vi "Write myRIO Data to the PI System via OMF (v1.0).vi"() -> ()   [LabVIEW 2014]
uses:
  <vilib>/Platform/TimedLoop/XDataNode/timing_clust.ctl
  <vilib>/Platform/TimedLoop/XDataNode/nitl_modes.ctl
  <vilib>/Platform/TimedLoop/XDataNode/wakeup.ctl
  <vilib>/myRIO/Instrument Drivers/Onboard Devices/Accelerometer/typedefs/Accelerometer Reference.ctl
  <vilib>/myRIO/Common/Instrument Driver Framework/Utilities/typedefs/myRIO Generic Hardware Reference.ctl
  <vilib>/myRIO/Common/Instrument Driver Framework/Utilities/typedefs/Hardware Version Enum.ctl
  <vilib>/myRIO/Common/Instrument Driver Framework/Utilities/typedefs/myRIO v1.0 Reference.ctl
  <vilib>/myRIO/Common/Instrument Driver Framework/Utilities/typedefs/Generic FPGA Reference.ctl
  <vilib>/myRIO/Common/Instrument Driver Framework/myRIO v1.0/Accelerometer/typedefs/Accelerometer Channels List.ctl
  <vilib>/myRIO/Common/Instrument Driver Framework/myRIO v1.0/Accelerometer/typedefs/Accelerometer Channels Enum.ctl
  <vilib>/userdefined/High Color/nirio_resource_hc.ctl
  <vilib>/myRIO/Common/Instrument Driver Framework/Utilities/vis/Is FPGA Ref Available.vi
  <vilib>/myRIO/Common/Instrument Driver Framework/myRIO v1.0/Accelerometer/vis/myRIO v1.1 Open Accelerometer.vi
  <vilib>/myRIO/Instrument Drivers/Onboard Devices/Accelerometer/vis/Read.vi
  <vilib>/myRIO/Common/Instrument Driver Framework/Utilities/vis/Validate Channels.vi
  <vilib>/myRIO/Common/Instrument Driver Framework/myRIO v1.0/Accelerometer/vis/myRIO v1.0 Reserve Accelerometer.vi
  <vilib>/myRIO/Common/Instrument Driver Framework/myRIO v1.0/Resource Manager/vis/myRIO v1.0 Reserve Channel List.vi
  <vilib>/myRIO/Common/Instrument Driver Framework/myRIO v1.0/Accelerometer/vis/myRIO v1.0 Build MUX Configuration Accelerometer.vi
  <vilib>/myRIO/Common/Instrument Driver Framework/myRIO v1.0/Resource Manager/vis/myRIO v1.0 Reserve Channel.vi
  <vilib>/myRIO/Common/Instrument Driver Framework/myRIO v1.0/Resource Manager/vis/myRIO v1.0 Unreserve Channel.vi
  <vilib>/myRIO/Common/Instrument Driver Framework/myRIO v1.0/Resource Manager/vis/myRIO v1.0 Build Mutex Name.vi
  <vilib>/Utility/VariantDataType/GetNumericInfo.vi
  <vilib>/Utility/error.llb/Error Cluster From Error Code.vi
  <vilib>/myRIO/Common/Instrument Driver Framework/myRIO v1.0/myRIO v1.1 Open.vi
  <vilib>/myRIO/Common/Instrument Driver Framework/myRIO v1.0/Accelerometer/vis/myRIO v1.0 Get Scaling Constant Accelerometer.vi
  <vilib>/myRIO/Common/Instrument Driver Framework/Utilities/vis/IO Manager.vi
  <vilib>/myRIO/Common/Instrument Driver Framework/Utilities/vis/Configuration Manager.vi
  <vilib>/myRIO/Common/Instrument Driver Framework/myRIO v1.0/myRIO v1.0 Close.vi
  <vilib>/myRIO/Common/Instrument Driver Framework/myRIO v1.0/Accelerometer/vis/myRIO v1.0 Read Accelerometer.vi
  <vilib>/platform/TimedLoop/XDataNode/XDataNode.xnode
  <vilib>/myRIO/Express VI/Onboard Devices/Accelerometer/Accelerometer Express VI.xnode
  <vilib>/myRIO/Instrument Drivers/Onboard Devices/Accelerometer/vis/myRIO Accelerometer Open.xnode
  <vilib>/Platform/TimedLoop/XDataNode/XDNodeRunTimeDep.lvlib
  <vilib>/myRIO/Instrument Drivers/Onboard Devices/Accelerometer/Accelerometer.lvlib
panel:
  out "Acceleration":T1(graph)
  in  "Stop looping":bool
  in  "OMF Static Type Instance Name":string="LabVIEW myRIO AF Element 3"
  out "Response body for initial OMF messages":string
  out "Reponse headers for initial OMF messages":string
  out "Number of continuous OMF data messages sent":i32
  out "Reponse body for continuous OMF data messages":string
  out "Response headers for continuous OMF data messages":string
  out "error out":errorcluster
  in  "Allow untrusted certificates?":bool=TRUE
  in  "OMF Dynamic Type Property Names and Formats":T2(array[cluster])=[{"Dynamic Property Name"="X acceleration", "Dynamic Property Format"=enum."number"}, {"Dynamic Property Name"="Y acceleration", "Dynamic Property Format"=enum."number"}, {"Dynamic Property Name"="Z acceleration", "Dynamic Property Format"=enum."number"}]
  in  "OMF Static Type Property Names, Formats, and Values":T3(array[cluster])=[{"Static Property Name"="Data ingress method", "Static Property Format"=enum."string", "Static Property Value"="\"OMF\""}]
  in  "Seconds in between continuous data messages":i32=1
  in  "OMF Static Type ID":string="LabVIEW myRIO Static Type 3"
  in  "OMF Dynamic Type ID":string="LabVIEW myRIO Dynamic Type 3"
  in  "OMF Container ID":string="LabVIEW myRIO Data Container 3"
  in  "OMF Producer Token":string="uid=034956ae-830c-4627-9778-e6724debe14b&crt=20180727152305511&sig=2y1S5b1wiy+iAvDMgQvLHble8CC54d+4WAt9WWHkGM8="
  in  "OMF Ingress URL":string="https://lopezpiserver:8118/ingress/messages"
  # "myRIO Accelerometer Data"
  # "Configuration"
  # "Response Messages"
  # "Note: if the response header is \"HTTP/1.1 204 No Content\" and the response body is empty, that indicates that a message was received successfully!"
  # "Note: the OMF Ingress URL and OMF Producer Token can be obtained from within the PI Data Collection Manager"
  # "(Stop sending continuous messages)"
  # "Note: If you are testing against a stock installation, one that still uses an untructed, self-signed certificate (which is the default), set this to \"ON\""
  # "Note: the Static Type Instance Name (below) will be the name of the PI AF Element that is created on the target PI System"
  # "Error Messages"
  # "Note: when specifying the value for a static property (above), if the property format is \"string\" add double quotes around the string value; if the property format \"number\", do not add double quotes around the numeric value."
  # "Note: remember the order in which you specify these dynamic properties! Later within your VI, you will wire in a string array of live data values for these dynamic properties, and the order of values in that array must match the order of properties that you specify above (i.e., if you listed that the first property is \"X acceleration\", you need to make sure that the first value in your string array is the x acceleration value)."
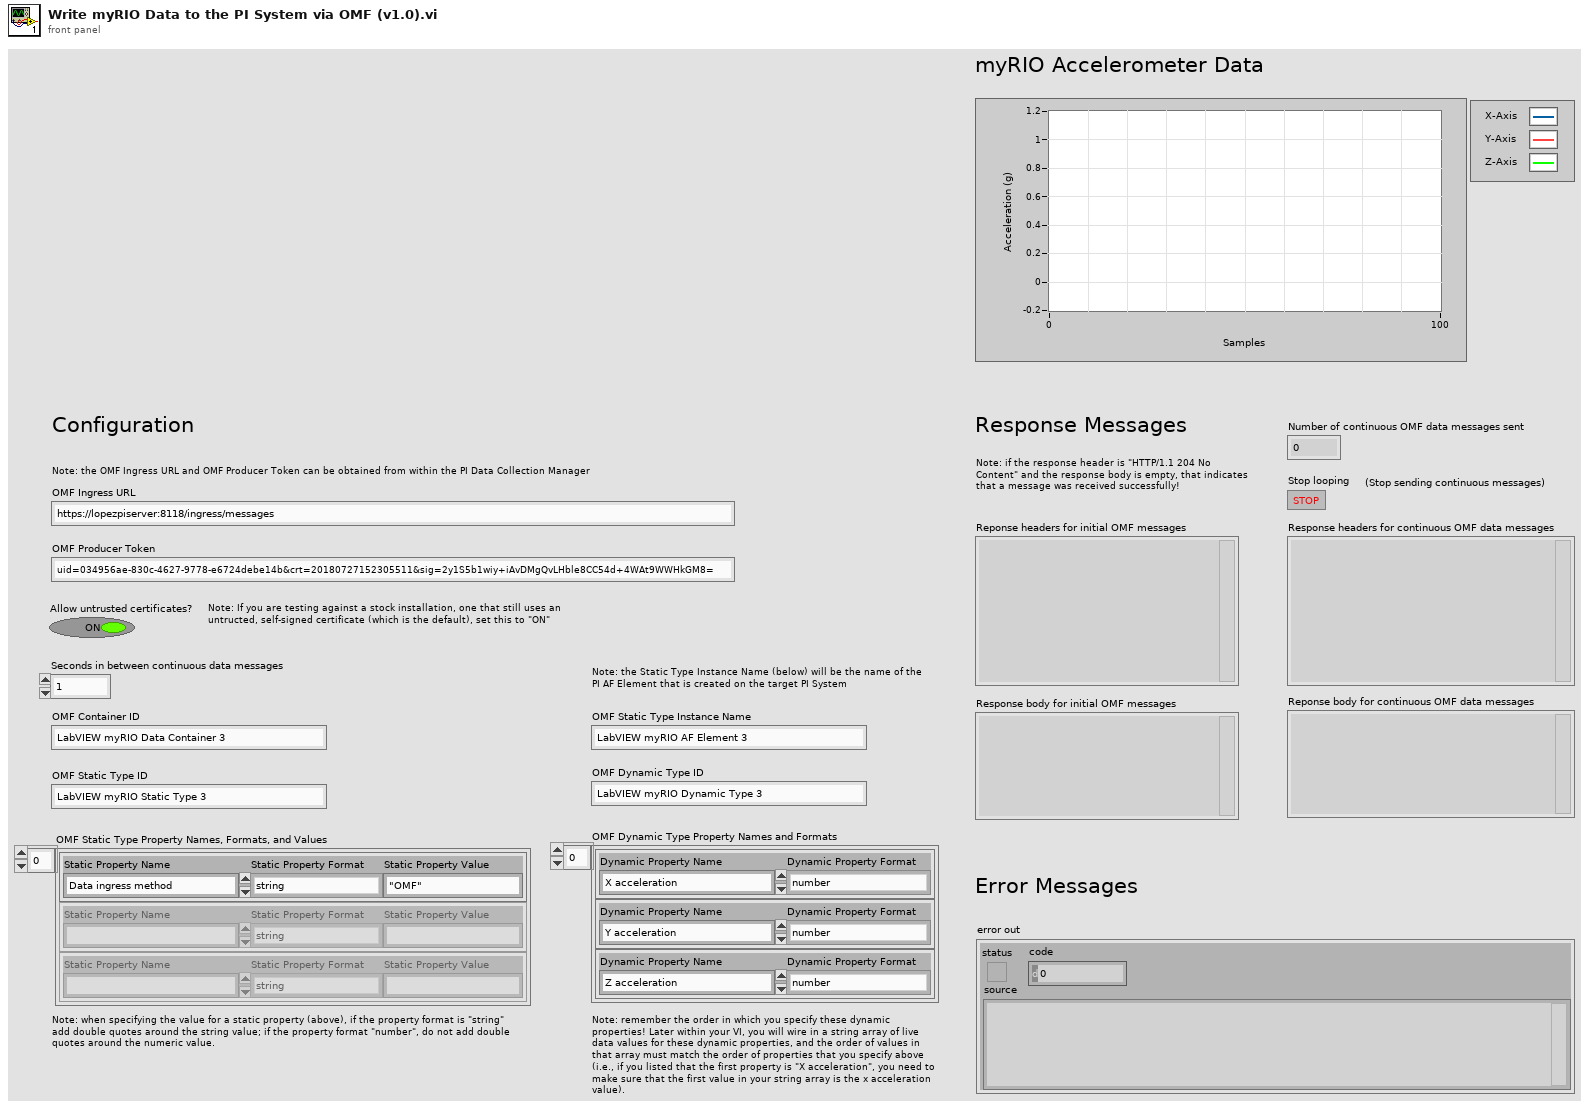
[diagram p1: front panel]
types:
  T1 = cluster{"X-Axis":dbl, "Y-Axis":dbl, "Z-Axis":dbl}
  T2 = cluster{"Dynamic Property Name":string, "Dynamic Property Format":enum16{"string", "number"}}[]
  T3 = cluster{"Static Property Name":string, "Static Property Format":enum16{"string", "number"}, "Static Property Value":string}[]
  T4 = typedef "LabVIEWHTTPClient.lvlib/ClientHandle.ctl" = refnum<k1>
  T5 = typedef "XDNodeRunTimeDep.lvlib/timing_clust.ctl" = cluster{"Expected End [f-1]":u64, "Actual End [f-1]":u64, "Finished Late? [f-1]":bool, "Expected End [i-1]":u64, "Actual End [i-1]":u64, "Finished Late? [i-1]":bool, "Expected Start [i]":u64, "Actual Start [i]":u64, "Expected Start [f]":u64, "Actual Start [f]":u64, "Source Name":string, "Structure Name":string, "Period":i64, "Deadline":i64, "Offset":i64, "Start":i64, "Priority":i32, "Timeout":i32, "Mode":T6, "Wakeup Reason":T7, "Error":errorcluster, "Source Type":string, "Secondary Source Type":string, "Global End Time":u64, "Global Start Time":u64, "Frame Duration":u64, "Iteration Duration":u64, "Assigned CPU":i32, "I/O Scan Engine Mode":u32}
  T6 = typedef "XDNodeRunTimeDep.lvlib/nitl_modes.ctl" = enum32{"No Change", "Process missed periods, maintain original phase", "Discard missed periods, maintain original phase", "Process missed periods, ignore original phase", "Discard missed periods, ignore original phase"}
  T7 = typedef "XDNodeRunTimeDep.lvlib/wakeup.ctl" = enum32{"Normal", "Aborted", "Asynchronous wakeup", "Timing source error", "Timed loop error", "Timeout"}
  T8 = typedef "Accelerometer.lvlib/Accelerometer Reference.ctl" = cluster{"myRIO Reference":T9, "Accelerometer Channels List":T13, "LSB Weight":dbl}
  T9 = typedef "myRIO Generic Hardware Reference.ctl" = cluster{"myRIO Model":T10, "myRIO Hardware Reference":T11}
  T10 = typedef "Hardware Version Enum.ctl" = enum16{"Unknown", "myRIO-1900", "myRIO-1950"}
  T11 = typedef "myRIO v1.0 Reference.ctl" = cluster{"Generic FPGA Reference":T12, "Allow multiple opens":bool}
  T12 = typedef "Generic FPGA Reference.ctl" = refnum<k20>
  T13 = typedef "Accelerometer Channels List.ctl" = T14[]
  T14 = typedef "Accelerometer Channels Enum.ctl" = enum16{"Not Connected", "X-Axis", "Y-Axis", "Z-Axis"}
  T15 = typedef "nirio_resource_hc.ctl" = tag
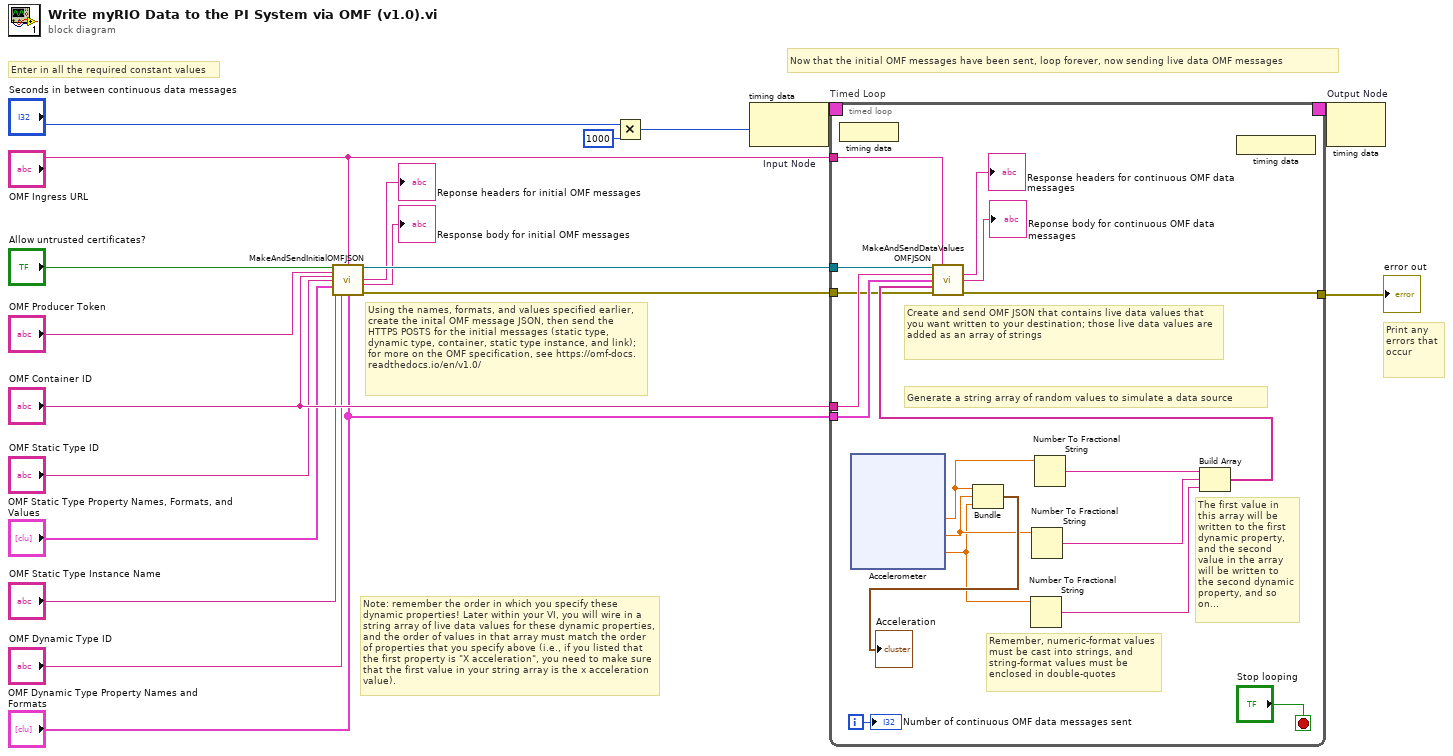
[diagram p0: block diagram]
diagram:
  # "Note: remember the order in which you specify these dynamic properties! Later within your VI, you will wire in a string array of live data values for these dynamic properties, and the order of values in that array must match the order of properties that you specify above (i.e., if you listed that the first property is \"X acceleration\", you need to make sure that the first value in your string array is the x acceleration value)."
  # "Now that the initial OMF messages have been sent, loop forever, now sending live data OMF messages"
  # "Using the names, formats, and values specified earlier, create the inital OMF message JSON, then send the HTTPS POSTS for the initial messages (static type, dynamic type, container, static type instance, and link); for more on the OMF specification, see https://omf-docs.readthedocs.io/en/v1.0/"
  # "Print any errors that occur"
  # "Enter in all the required constant values"
  n1 = call "MakeAndSendInitialOMFJSON.vi"("Allow untrusted certificates?"="Allow untrusted certificates?", "OMF Producer Token"="OMF Producer Token", "OMF Ingress URL"="OMF Ingress URL", "OMF Container ID"="OMF Container ID", "OMF Static Type ID"="OMF Static Type ID", "OMF Static Type Property Names, Formats, and Values"="OMF Static Type Property Names, Formats, and Values", "OMF Static Type Instance Name"="OMF Static Type Instance Name", "OMF Dynamic Type ID"="OMF Dynamic Type ID", "OMF Dynamic Type Property Names and Formats"="OMF Dynamic Type Property Names and Formats") -> ("client handle out"=w10:T4, "Reponse headers for initial OMF messages"=→"Reponse headers for initial OMF messages":string, "Response body for initial OMF messages"=→"Response body for initial OMF messages":string, "error out"=w9:errorcluster)  [unwired: 3 in]
  n2 = Multiply(x="Seconds in between continuous data messages", y=1000) -> (x*y=w14:i32)
  n3 = node-c288 "Input Node"(w14) -> (w18:T5)
  n4 = timed-loop "Timed Loop" {
    timing: w18 -> [_]
    timing-out: [_] -> w17
    tunnel: w10 -> [w29]
    tunnel: "OMF Ingress URL" -> [w28]
    tunnel: w9 -> [w30]
    tunnel: [w25] -> w19
    tunnel: "OMF Container ID" -> [w32]
    tunnel: "OMF Dynamic Type Property Names and Formats" -> [w33]
    i -> [w37]
    stop <- "Stop looping" stop-if-true
    # "Remember, numeric-format values must be cast into strings, and string-format values must be enclosed in double-quotes"
    # "The first value in this array will be written to the first dynamic property, and the second value in the array will be written to the second dynamic property, and so on..."
    # "Generate a string array of random values to simulate a data source"
    # "Create and send OMF JSON that contains live data values that you want written to your destination; those live data values are added as an array of strings"
    n5 = node-c288 ("Output Node")() -> ()  [unwired: 1 in]
    n6 = xnode "Accelerometer"() -> ("X-Axis"=w22:dbl, "Y-Axis"=w21:dbl, "Z-Axis"=w20:dbl)  [unwired: 1 in, 1 out]
    n7 = Bundle("X-Axis"=w22, "Y-Axis"=w21, "Z-Axis"=w20) -> (→"Acceleration":T1)  [unwired: 1 in]
    n8 = Number To Fractional String(number=w20) -> (F-format string=w34:string)  [unwired: 3 in]
    n9 = Number To Fractional String(number=w21) -> (F-format string=w35:string)  [unwired: 3 in]
    n10 = Number To Fractional String(number=w22) -> (F-format string=w36:string)  [unwired: 3 in]
    n11 = Build Array "Build Array"(w36, w35, w34) -> (w31:string[])
    n12 = call "MakeAndSendDataValuesOMFJSON.vi"("client handle"=w29, "OMF Ingress URL"=w28, "OMF Container ID"=w32, "OMF Dynamic Type Property Names and Formats"=w33, "Array of Values"=w31, "error in (no error)"=w30) -> ("Response headers for continuous OMF data messages"=→"Response headers for continuous OMF data messages":string, "Reponse body for continuous OMF data messages"=→"Reponse body for continuous OMF data messages":string, "error out"=w25:errorcluster)  [unwired: 7 in]
    n13 = node-c288() -> ()  [unwired: 1 out]
    "Number of continuous OMF data messages sent" <- w37
  }
  "error out" <- w19
  n14 = node-c288 "Output Node"(w17) -> ()  [unwired: 1 out]
